vi "Secondary System.vi"() -> (2 "Arm Height Setting":dbl)   [LabVIEW 2013]
panel:
  in  "Arm Constants":T1={"Top Center Peg"=166.0, "Top Outer Pegs"=155.0, "Middle Center Peg"=118.0, "Middle Outer Pegs"=109.0, "Lower Center Peg"=76.0, "Lower Outside Pegs"=73.0, "Feed"=20.0, "Floor"=13.0}
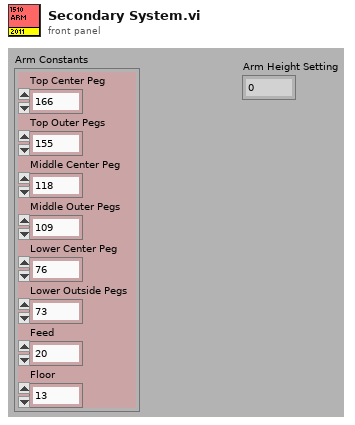
[diagram p1: front panel]
types:
  T1 = cluster{"Top Center Peg":dbl, "Top Outer Pegs":dbl, "Middle Center Peg":dbl, "Middle Outer Pegs":dbl, "Lower Center Peg":dbl, "Lower Outside Pegs":dbl, "Feed":dbl, "Floor":dbl}
  T2 = typedef "Arm Joystick.ctl" = cluster{"Buttons":T3, "Axes":cluster{"axis 1 (x)":dbl, "axis 2 (y)":dbl, "axis 3 (throttle)":dbl, "axis 4":dbl, "axis 5":dbl, "axis 6":dbl}}
  T3 = typedef "WPI_JoystickButtonState.ctl" = cluster{"Button 1":bool, "Button 2":bool, "Button 3":bool, "Button 4":bool, "Button 5":bool, "Button 6":bool, "Button 7":bool, "Button 8":bool, "Button 9":bool, "Button 10":bool, "Button 11":bool, "Button 12":bool}
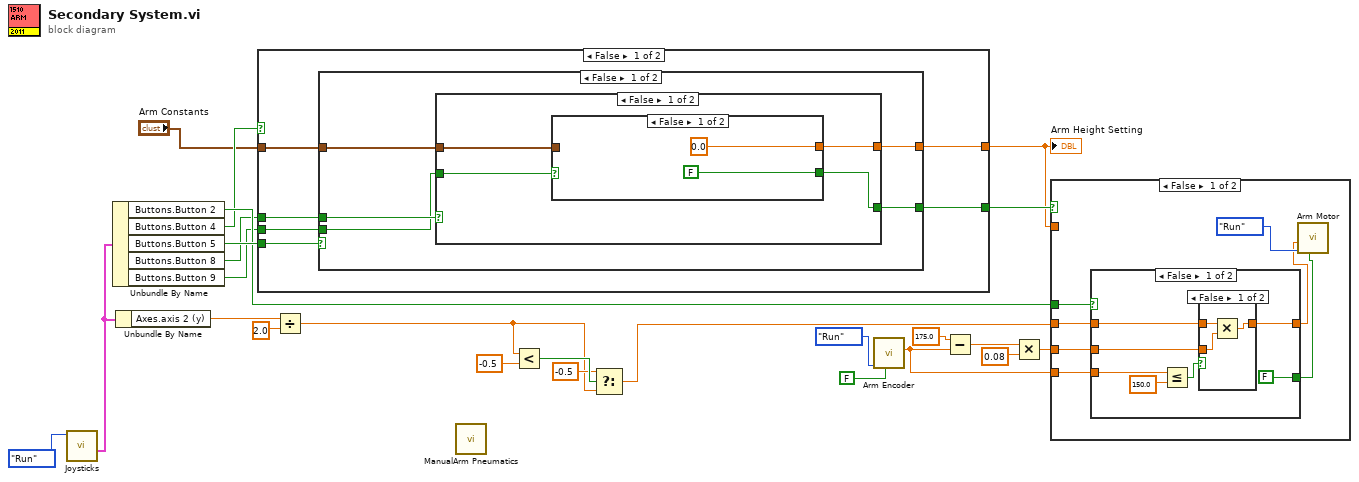
[diagram p0: block diagram]
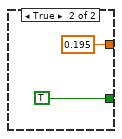
[diagram p3: hidden frame]
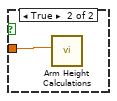
[diagram p4: hidden frame]
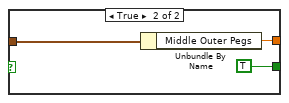
[diagram p5: hidden frame]
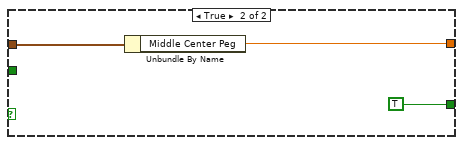
[diagram p6: hidden frame]
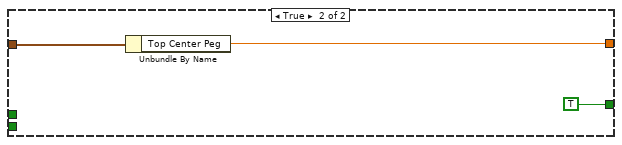
[diagram p7: hidden frame]
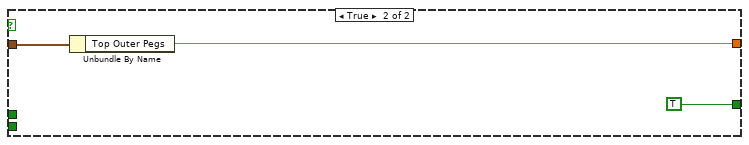
[diagram p8: hidden frame]
diagram:
  n1 = call "Joysticks.vi"("Mode"=enum16{"Init", "Run", "End"}."Run") -> ("Arm Joystick"=w22:T2)  [unwired: 8 out]
  n2 = Unbundle By Name(w22) -> ("Buttons.Button 2"=w14:bool, "Buttons.Button 4"=w10:bool, "Buttons.Button 5"=w24:bool, "Buttons.Button 8"=w11:bool, "Buttons.Button 9"=w12:bool)
  n3 = Unbundle By Name(w22) -> ("Axes.axis 2 (y)"=w15:dbl)
  n4 = case shown="False" w10 {
    tunnel: [w29 TRUE] -> w13
    tunnel: [w30 w51] -> w9
    tunnel: w24 -> [w28 _]
    tunnel: w11 -> [w27 _]
    tunnel: w12 -> [w26 _]
    tunnel: "Arm Constants" -> [w25 w52]
    frame False {
      n5 = case shown="False" w28 {
        tunnel: [w34 w49] -> w30
        tunnel: [w35 TRUE] -> w29
        tunnel: w27 -> [w33 _]
        tunnel: w26 -> [w32 _]
        tunnel: w25 -> [w31 w48]
        frame False {
          n6 = case shown="False" w33 {
            tunnel: [w39 TRUE] -> w35
            tunnel: [w38 w45] -> w34
            tunnel: w32 -> [w37 _]
            tunnel: w31 -> [w36 w46]
            frame False {
              n7 = case shown="False" w37 {
                tunnel: [FALSE TRUE] -> w39
                tunnel: [0.0 ("Middle Outer Pegs") w42] -> w38
                tunnel: w36 -> [_ w43]
                frame False {
                }
                frame True {
                  n8 = Unbundle By Name(w43) -> ("Middle Outer Pegs"=w42:dbl)
                }
              }
            }
            frame True {
              n9 = Unbundle By Name(w46) -> ("Middle Center Peg"=w45:dbl)
            }
          }
        }
        frame True {
          n10 = Unbundle By Name(w48) -> ("Top Center Peg"=w49:dbl)
        }
      }
    }
    frame True {
      n11 = Unbundle By Name(w52) -> ("Top Outer Pegs"=w51:dbl)
    }
  }
  "Arm Height Setting" <- w9
  n12 = Divide(x=w15, y=2.0) -> (x/y=w3:dbl)
  n13 = call "ManualArm Pneumatics.vi"() -> ()  [unwired: 1 out]
  n14 = Less?(x=w3, y=-0.5) -> (x < y?=w5:bool)
  n15 = Select(t=-0.5, s=w5, f=w3) -> (s? t:f=w2:dbl)
  n16 = call "Arm Encoder.vi"("Reset Encoder?"=FALSE, "Mode"=enum16{"Init", "Run", "End"}."Run") -> ("Get Arm Encoder"=w8:dbl)  [unwired: 1 in, 8 out]
  n17 = Subtract(x=175.0, y=w8) -> (x-y=w16:dbl)
  n18 = Multiply(x=w16, y=0.08) -> (x*y=w18:dbl)
  n19 = case shown="False" w13 {
    tunnel: w14 -> [w57 _]
    tunnel: w8 -> [w60 _]
    tunnel: w2 -> [w59 _]
    tunnel: w18 -> [w58 _]
    tunnel: w9 -> [_ w74]
    frame False {
      n20 = case shown="False" w57 {
        tunnel: w60 -> [w67 _]
        tunnel: w59 -> [w65 _]
        tunnel: w58 -> [w64 _]
        tunnel: [w63 0.195] -> w55
        tunnel: [FALSE TRUE] -> w54
        frame False {
          n21 = Less Or Equal?(x=w67, y=150.0) -> (x <= y?=w66:bool)
          n22 = case shown="False" w66 {
            tunnel: w65 -> [w70 w71]
            tunnel: [w68 w71] -> w63
            tunnel: w64 -> [w69 _]
            frame False {
              n23 = Multiply(x=w70, y=w69) -> (x*y=w68:dbl)
            }
            frame True {
            }
          }
        }
        frame True {
        }
      }
      n24 = call "Arm Motor.vi"("Stall Arm?"=w54, "Mode"=enum16{"Init", "Run", "End"}."Run", "Arm motor speed"=w55) -> ()  [unwired: 1 in, 8 out]
    }
    frame True {
      n25 = call "Arm Height Calculations.vi"("Height Input"=w74) -> ()  [unwired: 11 out]
    }
  }
